vi "_localizeDataPluginMessage.vi"(11 "message in":T1) -> (3 "message out":string)   [LabVIEW 2020]
uses:
  <vilib>/Platform/storage/utility/DataPluginSynchronization/_localizeDataPluginMessageEnum.ctl
panel:
  in  "message table out":string[](array[string])=["Installed", "Not Installed", "Update Available", "Latest version: ", "Double-click the description to find further information on the National Instruments website.", "Install/Update DataPlugins", "Offline: ", "LabVIEW can not find any DataPlugins on web.\nPlease ensure that your network connection is working.\nFor the following dialog box, you cannot install or update DataPlugins.", "No updates found. Your DataPlugins are up-to-date.", "Loading DataPlugins from ni.com/dataplugins", "Downloading the installer and installing the DataPlugins on the computer", "Install", "Update", "Succeed", "Failed", "Installation successful.", "Begin with *. to search for file extension only", "Current version: ", "Failed to install the DataPlugin. \n\nPossible reasons include a failed network connection or a server connection problem.\n\nLabVIEW closes this dialog box after you click the OK button.", "Downloading the installer and installing update", "Update successful.", "Failed to update the DataPlugin.\n\nPossible reasons include a failed network connection or a server connection problem.\n\nLabVIEW closes this dialog box after you click the OK button.", "Updated", "Failed to update DataPlugins.\n\nPossible reasons include a failed network connection or a server connection problem.\n\nLabVIEW closes this dialog box after you click the OK button."]
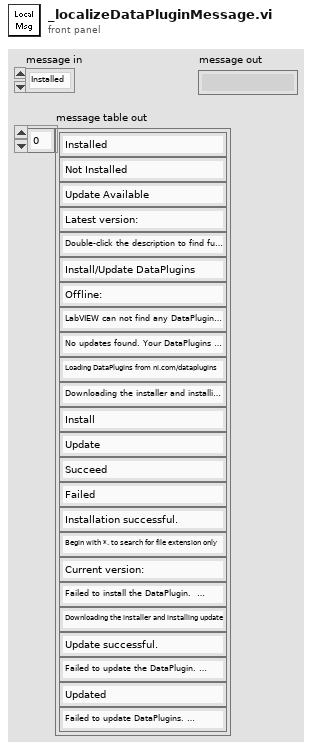
[diagram p1: front panel]
types:
  T1 = typedef "_localizeDataPluginMessageEnum.ctl" = enum16{"Installed", "Not Installed", "Updates Available", "Latest version:", "Double click the \"Description\" cell.", "Install/Update DataPlugins", "Offline: ", "Please ensure that your network connection is working.", "No DataPlugins can be updated.", "Loading DataPlugins from ni.com/dataplugins", "Acquiring and installing ", "Install", "Update", "Succeed", "Failed", " Installation successful.", "Include *. to search for a file extension", "Current version:", " Installation failed.", "Installing update", "Update successful.", "Update failed.", "Updated", "Failed to update DataPlugins."}
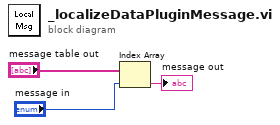
[diagram p0: block diagram]
diagram:
  n1 = Index Array(array="message table out", index="message in") -> (element=→"message out":string)
